vi "Exam.vi"() -> ()   [LabVIEW 2018]
panel:
  in  "정지":bool
  in  "추가숫자":dbl
  out "배열":dbl[](array[numeric])
  in  "추가":bool
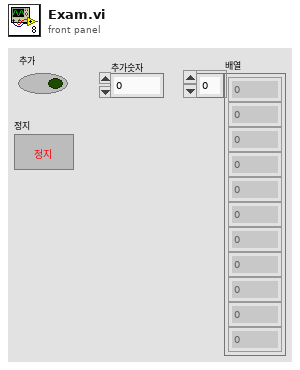
[diagram p1: front panel]
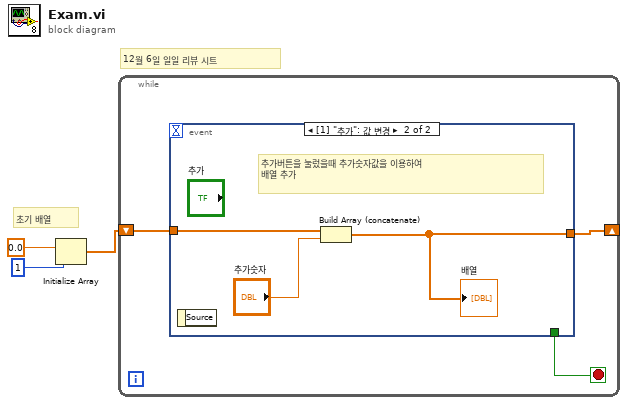
[diagram p0: block diagram]
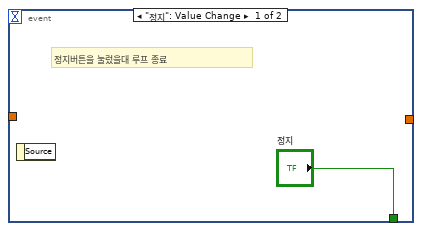
[diagram p2: hidden frame]
diagram:
  # "초기 배열"
  # "12월 6일 일일 리뷰 시트"
  n1 = Initialize Array(0.0 ("원소"), 1 ("차원 크기")) -> (w1:dbl[])
  n2 = while {
    shift-right: [w4] -> _
    shift-left: w1 -> [w5]
    stop <- w6 stop-if-true
    n3 = event shown="[1] \"추가\": 값 변경" {
      selector: _ -> [_ _]
      dyn-events: _ -> [_ _]
      timeout: _ -> [_ _]
      tunnel: ["정지" _] -> w6
      tunnel: w5 -> [_ w10]
      tunnel: [_ w8] -> w4
      event "정지": Value Change {
        # "정지버튼을 눌렀을대 루프 종료"
        n4 = event-data() -> ()  [unwired: 1 in, 1 out]
      }
      event "추가": Value Change {
        # "추가버튼을 눌렀을때 추가숫자값을 이용하여\n배열 추가"
        n5 = event-data() -> ()  [unwired: 1 in, 1 out]
        n6 = Build Array (concatenate)(w10, "추가숫자") -> (w8:dbl[])
        "배열" <- w8
      }
    }
  }
